vi "camera demo.vi"() -> ()   [LabVIEW 2014]
uses:
  <vilib>/userdefined/High Color/IMAQdx.ctl
  <vilib>/vision/driver/NI_Vision_Acquisition_Software.lvlib
panel:
  out "error out":errorcluster
  in  "Webcam":T1
  out "Color Image":T2(plugin-control)
  out "BW Image":T2(plugin-control)
  out "Nb Circles":i32
  out "Camera Data":T3(array[cluster])
  in  "stop robot control":bool
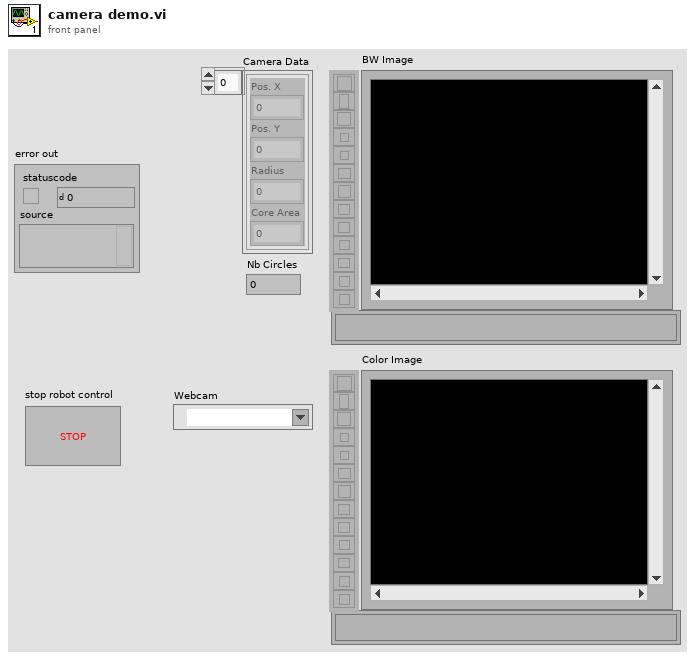
[diagram p1: front panel]
types:
  T1 = typedef "IMAQdx.ctl" = refnum<k21>
  T2 = typedef "IMAQ Image.ctl" = refnum<image>
  T3 = cluster{"Pos. X":i32, "Pos. Y":i32, "Radius":i32, "Core Area":i32}[]
  T4 = typedef "Image Type" = u32
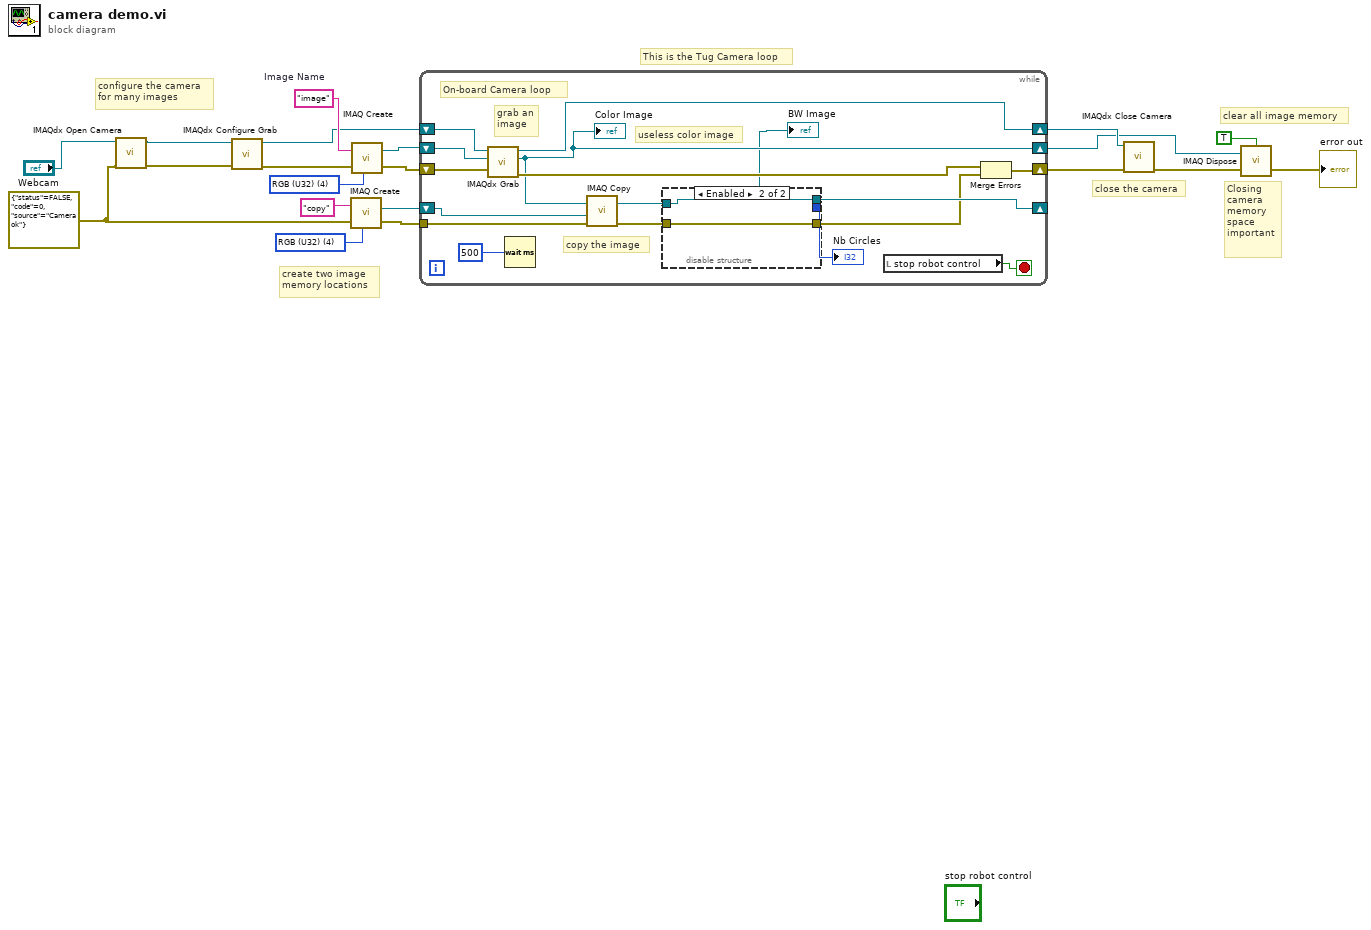
[diagram p0: block diagram]
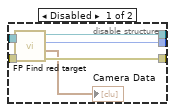
[diagram p2: hidden frame]
diagram:
  w19 = T4 4 items=["Grayscale (U8)", "Grayscale (I16)", "Grayscale (SGL)", "Complex (CSG)", "RGB (U32)", "HSL (U32)", "RGB (U64)", "Grayscale (U16)"] ("Image Type")
  w5 = errorcluster {"status"=FALSE, "code"=0, "source"="Camera ok"} ("error in")
  w17 = T4 4 items=["Grayscale (U8)", "Grayscale (I16)", "Grayscale (SGL)", "Complex (CSG)", "RGB (U32)", "HSL (U32)", "RGB (U64)", "Grayscale (U16)"] ("Image Type")
  w18 = "image"  # Image Name
  # "create two image\nmemory locations"
  # "Closing \ncamera\nmemory\nspace\nimportant"
  # "This is the Tug Camera loop"
  # "clear all image memory"
  # "close the camera"
  # "configure the camera\nfor many images"
  n1 = call <vilib>:"IMAQdx Open Camera.vi"("error in"=w5, "Session In"="Webcam") -> ("error out"=w3:errorcluster, "Session Out"=w4:T1)  [unwired: 8 in]
  n2 = call <vilib>:"IMAQdx Configure Grab.vi"("error in"=w3, "Session In"=w4) -> ("error out"=w16:errorcluster, "Session Out"=w13:T1)  [unwired: 8 out]
  n3 = call "IMAQ Create"("Image Name"="copy", "Image Type"=w19, "error in (no error)"=w5) -> ("New Image"=w10:T2, "error out"=w9:errorcluster)  [unwired: 2 in]
  n4 = call "IMAQ Create"("Image Name"=w18, "Image Type"=w17, "error in (no error)"=w16) -> ("New Image"=w12:T2, "error out"=w11:errorcluster)  [unwired: 1 in, 1 out]
  n5 = while {
    shift-right: [w29] -> w6
    shift-left: w11 -> [w27]
    shift-right: [w28] -> w7
    shift-left: w12 -> [w36]
    shift-right: [w31] -> w8
    shift-left: w13 -> [w35]
    tunnel: w9 -> [w33]
    shift-right: [w24] -> _
    shift-left: w10 -> [w32]
    stop <- w21 stop-if-true
    # "useless color image"
    # "grab an\nimage"
    # "copy the image"
    # "On-board Camera loop"
    n6 = call <vilib>:"IMAQdx Grab.vi"("error in"=w27, "Image In"=w36, "Session In"=w35) -> ("error out"=w30:errorcluster, "Image Out"=w28:T2, "Session Out"=w31:T1)  [unwired: 5 in, 1 out]
    "Color Image" <- w28
    n7 = Wait (ms)(milliseconds to wait=u32 500) -> ()  [unwired: 1 out]
    n8 = call "IMAQ Copy"("error in (no error)"=w33, "Image Dst"=w32, "Image Src"=w28) -> ("error out"=w25:errorcluster, "Image Dst Out"=w26:T2)  [unwired: 3 in]
    n9 = disable-structure shown="Enabled" {
      disable-tunnel: w26 -> [w42 w43]
      disable-tunnel: w25 -> [w41 w44]
      disable-tunnel: [w40 w43] -> w24
      disable-tunnel: [w39 w44] -> w23
      disable-tunnel: [w38 _] -> w22
      frame Disabled {
        n10 = call "FP Find red target.vi"("Image In"=w42, "error in (no error)"=w41) -> ("Image Dst Out"=w40:T2, "Nb Circles (Circle Detection 1)"=w38:i32, "Camera Data"=→"Camera Data":T3, "error out"=w39:errorcluster)
      }
      frame Enabled {
      }
    }
    "BW Image" <- w24
    "Nb Circles" <- w22
    n11 = local read "stop robot control"() -> (w21:bool)
    n12 = Merge Errors(w30, w23) -> (w29:errorcluster)
  }
  n13 = call <vilib>:"IMAQdx Close Camera.vi"("error in"=w6, "Session In"=w8) -> ("error out"=w14:errorcluster)  [unwired: 9 out]
  n14 = call "IMAQ Dispose"("All Images? (No)"=TRUE, "Image"=w7, "error in (no error)"=w14) -> ("error out"=→"error out":errorcluster)  [unwired: 3 out]
